vi "ep_Process data (N Samples).vi"(7 "timestamps":timestamp[](array[timestamp]), 8 "error in":errorcluster, 9 "digital data":bool[][](array[boolean]), 10 "analog data":dbl[][](array[numeric]), 11 "task in":T1={"file refnums"=[], "Data Object"=refnum, "config info"={"station_name"="", "rec_dev_id"="", "rev_year"=1999.0, "TT"=0, "##A"=0, "##D"=0, "analog channel info"=[], "status channel info"=[], "lf"=-inf, "nrates"=65535, "samp info"=[], "initial timestamp"=timestamp(0 s since 1904-01-01), "trigger timestamp"=timestamp(0 s since 1904-01-01), "ft"=enum."Binary", "timemult"=1.0}, "public inf content"={"Source"="", "Record Type"=enum."Fault", "Phase ID"="", "Event Description"="", "Device ID"="", "Distance of Fault"=-1.0, "Distance Unit"=enum."Miles", "Max_Current"=inf, "Min_Current"=-inf, "Max_Voltage"=inf, "Min_Voltage"=-inf, "EventNoteCount"=0, "Event Information"=[]}, "private inf content"=[], "internal buffers"={"start index"=1, "config to public inf"=enum."disabled", "static config info"="", "static file_des record inf"="", "static file_des channel inf"="", "public inf"="", "private inf"=""}} {"public inf content"."Event Information"."min sample number" max=9999999999; "public inf content"."Event Information"."max sample number" max=9999999999; "config info"."nrates" max=999; "config info"."status channel info"."Dn" min=1 max=999999; "config info"."analog channel info"."An" min=1 max=999999; "config info"."trigger timestamp" format="%<%H:%M:%S%6u\n%d/%m/%Y>T"; "config info"."initial timestamp" format="%<%H:%M:%S%6u\n%d/%m/%Y>T"; "config info"."##D" max=999999; "config info"."##A" max=999999; "config info"."TT" min=1 max=999999; "config info"."rev_year" min=1999.0 max=1999.0}) -> (0 "error out":errorcluster, 1 "digital data out":u16[][](array[numeric]), 2 "analog data out":u16[][](array[numeric]), 3 "dup task":T1={"file refnums"=[], "Data Object"=refnum, "config info"={"station_name"="", "rec_dev_id"="", "rev_year"=1999.0, "TT"=0, "##A"=0, "##D"=0, "analog channel info"=[], "status channel info"=[], "lf"=-inf, "nrates"=65535, "samp info"=[], "initial timestamp"=timestamp(0 s since 1904-01-01), "trigger timestamp"=timestamp(0 s since 1904-01-01), "ft"=enum."Binary", "timemult"=1.0}, "public inf content"={"Source"="", "Record Type"=enum."Fault", "Phase ID"="", "Event Description"="", "Device ID"="", "Distance of Fault"=-1.0, "Distance Unit"=enum."Miles", "Max_Current"=inf, "Min_Current"=-inf, "Max_Voltage"=inf, "Min_Voltage"=-inf, "EventNoteCount"=0, "Event Information"=[]}, "private inf content"=[], "internal buffers"={"start index"=1, "config to public inf"=enum."disabled", "static config info"="", "static file_des record inf"="", "static file_des channel inf"="", "public inf"="", "private inf"=""}} {"public inf content"."Event Information"."min sample number" max=9999999999; "public inf content"."Event Information"."max sample number" max=9999999999; "config info"."nrates" max=999; "config info"."status channel info"."Dn" min=1 max=999999; "config info"."analog channel info"."An" min=1 max=999999; "config info"."trigger timestamp" format="%<%H:%M:%S%6u\n%d/%m/%Y>T"; "config info"."initial timestamp" format="%<%H:%M:%S%6u\n%d/%m/%Y>T"; "config info"."##D" max=999999; "config info"."##A" max=999999; "config info"."TT" min=1 max=999999; "config info"."rev_year" min=1999.0 max=1999.0}, 4 "data length":i32, 5 "timestamps out":u32[](array[numeric]))   [LabVIEW 2011, in "NI_EP_COMTRADE.lvlib"]
uses:
  <vilib>/addons/Electrical Power/File IO/NI_EP_COMTRADE.lvlib
  <vilib>/addons/Electrical Power/File IO/COMTRADE/typedefs/ep_Task.ctl
  <vilib>/addons/Electrical Power/File IO/COMTRADE/typedefs/ep_Config Info.ctl
  <vilib>/addons/Electrical Power/File IO/COMTRADE/typedefs/ep_Analog Channel Info.ctl
  <vilib>/addons/Electrical Power/File IO/COMTRADE/typedefs/ep_Status Channel Info.ctl
  <vilib>/addons/Electrical Power/File IO/COMTRADE/typedefs/ep_File Format.ctl
  <vilib>/addons/Electrical Power/File IO/COMTRADE/typedefs/ep_Public Inf Content.ctl
  <vilib>/addons/Electrical Power/File IO/COMTRADE/typedefs/ep_Public Event Inf.ctl
  <vilib>/addons/Electrical Power/File IO/COMTRADE/typedefs/ep_Private Inf Content.ctl
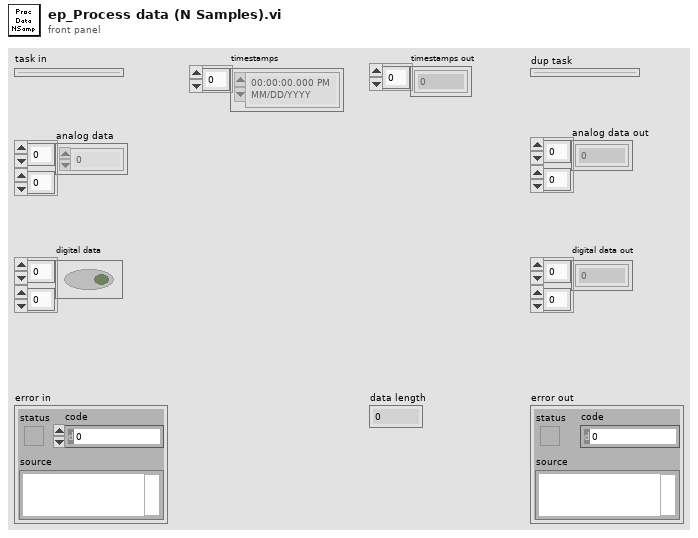
[diagram p1: front panel]
types:
  T1 = typedef "NI_EP_COMTRADE.lvlib/ep_Task.ctl" = cluster{"file refnums":refnum<file>[], "Data Object":refnum<k20>, "config info":T2, "public inf content":T6, "private inf content":T8, "internal buffers":cluster{"start index":u32, "config to public inf":enum16{"disabled", "enabled", "buffered"}, "static config info":string, "static file_des record inf":string, "static file_des channel inf":string, "public inf":string, "private inf":string}}
  T2 = typedef "NI_EP_COMTRADE.lvlib/ep_Config Info.ctl" = cluster{"station_name":string, "rec_dev_id":string, "rev_year":dbl, "TT":u32, "##A":u32, "##D":u32, "analog channel info":T3[], "status channel info":T4[], "lf":sgl, "nrates":u16, "samp info":cluster{"samp":sgl, "endsamp":u32}[], "initial timestamp":timestamp, "trigger timestamp":timestamp, "ft":T5, "timemult":sgl}
  T3 = typedef "NI_EP_COMTRADE.lvlib/ep_Analog Channel Info.ctl" = cluster{"An":u32, "ch_id":string, "ph":string, "ccbm":string, "uu":string, "a":sgl, "b":sgl, "skew":sgl, "min":i32, "max":i32, "primary":sgl, "secondary":sgl, "PS":enum16{"P", "S"}}
  T4 = typedef "NI_EP_COMTRADE.lvlib/ep_Status Channel Info.ctl" = cluster{"Dn":u32, "ch_id":string, "ph":string, "ccbm":string, "Y":bool}
  T5 = typedef "NI_EP_COMTRADE.lvlib/ep_File Format.ctl" = enum16{"ASCII", "Binary"}
  T6 = typedef "NI_EP_COMTRADE.lvlib/ep_Public Inf Content.ctl" = cluster{"Source":string, "Record Type":enum16{"Fault", "Unknown", "Misoperation", "Close", "Trip", "Reclose", "Power swing", "Simulation"}, "Phase ID":string, "Event Description":string, "Device ID":string, "Distance of Fault":dbl, "Distance Unit":enum16{"Miles", "Kilometers", "Percent of line", "Percent of setting", "Ohms"}, "Max_Current":dbl, "Min_Current":dbl, "Max_Voltage":dbl, "Min_Voltage":dbl, "EventNoteCount":u32, "Event Information":T7[]}
  T7 = typedef "NI_EP_COMTRADE.lvlib/ep_Public Event Inf.ctl" = cluster{"channel number":u32, "max value":dbl, "min value":dbl, "max sample number":u64, "min sample number":u64, "max sample text":string[], "min sample text":string[]}
  T8 = typedef "NI_EP_COMTRADE.lvlib/ep_Private Inf Content.ctl" = cluster{"Section Header":string, "Entry Names":string[], "Entry Values":string[]}[]
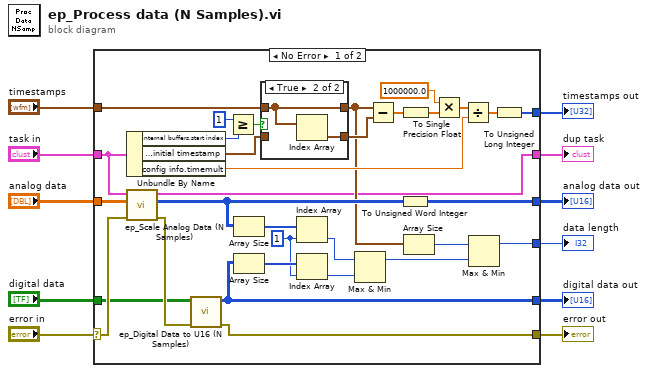
[diagram p0: block diagram]
diagram:
  n1 = case shown="No Error" "error in" {
    selector: "error in" -> [w34 w48]
    tunnel: "analog data" -> [w39 _]
    tunnel: "task in" -> [w31 w49]
    tunnel: [w13 w49] -> w8
    tunnel: "digital data" -> [w33 _]
    tunnel: [w36 w48] -> w7
    tunnel: [w23 _] -> w5
    tunnel: [w37 _] -> w4
    tunnel: [w32 _] -> w3
    tunnel: "timestamps" -> [w17 _]
    tunnel: [w14 _] -> w1
    frame No Error {
      w41 = 1 ("index")
      n2 = Unbundle By Name(w31) -> ("internal buffers.start index"=w22:u32, "config info.initial timestamp"=w19:timestamp, "config info.timemult"=w26:sgl)
      n3 = call <vilib>:"ep_Scale Analog Data (N Samples).vi"("error in"=w34, "analog data"=w39, "task in"=w31) -> ("error out"=w35:errorcluster, "scaled analog data"=w38:i16[][], "dup task"=w13:T1)  [unwired: 6 in]
      n4 = call <vilib>:"ep_Digital Data to U16 (N Samples).vi"("error in"=w35, "digital signal"=w33) -> ("error out"=w36:errorcluster, "U16 digital data"=w32:u16[][])  [unwired: 8 in]
      n5 = Greater Or Equal?(x=u32 1, y=w22) -> (x >= y?=w20:bool)
      n6 = Array Size(array=w38) -> (size(s)=w43:i32[])
      n7 = Array Size(array=w32) -> (size(s)=w42:i32[])
      n8 = case shown="True" w20 {
        tunnel: w19 -> [w45 _]
        tunnel: [w45 w46] -> w18
        tunnel: w17 -> [w44 w47]
        tunnel: [w44 w47] -> w16
        frame False {
        }
        frame True {
          n9 = Index Array(array=w47) -> (element=w46:timestamp)  [unwired: 1 in]
        }
      }
      n10 = Index Array(array=w43, index=w41) -> (element=w40:i32)
      n11 = Index Array(array=w42, index=w41) -> (element=w25:i32)
      n12 = Max & Min(x=w40, y=w25) -> (max(x,y)=w24:i32)  [unwired: 1 out]
      n13 = Subtract(x=w16, y=w18) -> (x-y=w30:dbl[])
      n14 = To Unsigned Word Integer(number=w38) -> (unsigned 16bit integer=w37:u16[][])
      n15 = To Single Precision Float(number=w30) -> (single precision float=w29:sgl[])
      n16 = Array Size(array=w16) -> (size(s)=w15:i32)
      n17 = Multiply(x=sgl 1000000.0, y=w29) -> (x*y=w28:sgl[])
      n18 = Divide(x=w28, y=w26) -> (x/y=w27:sgl[])
      n19 = Max & Min(x=w15, y=w24) -> (max(x,y)=w23:i32)  [unwired: 1 out]
      n20 = To Unsigned Long Integer(number=w27) -> (unsigned 32bit integer=w14:u32[])
    }
    frame Error {
    }
  }
  "error out" <- w7
  "dup task" <- w8
  "data length" <- w5
  "analog data out" <- w4
  "digital data out" <- w3
  "timestamps out" <- w1
